vi "lookup_node_predecessors.vi"(10 "node":refnum<class "Node.lvclass">, 11 "digraph":refnum<class "DiGraph.lvclass">) -> (1 "predecessors":refnum<class "Node.lvclass">[](array[class]), 2 "node not found?":bool)   [LabVIEW 2020, in "graph.lvlib" / "DiGraph.lvclass"]
uses:
  DiGraph.lvclass
  C:/Projects/labview-project-load-tools/source/submodules/graph-api-labview/source/api/Graph/Graph.lvclass
  Node/Node.lvclass
  Node/Node.lvclass/Node.ctl
  DiGraph.lvclass/DiGraph.ctl
  Graph/Graph.lvclass/Graph.ctl
  Graph/Graph.lvclass
  0d9acaa0-7633-4a41-a63c-eb8e9d282815.vi
  C:/Projects/labview-project-load-tools/source/submodules/graph-api-labview/source/api/DiGraph/DiGraph.lvclass
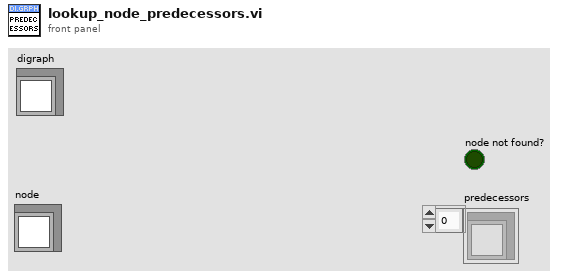
[diagram p1: front panel]
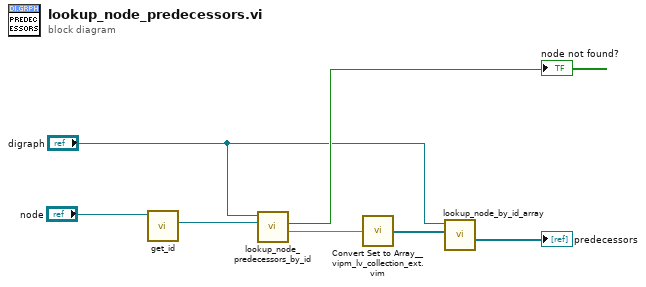
[diagram p0: block diagram]
diagram:
  n1 = call "get_id.vi"("node"="node") -> ("node-id"=w5:refnum<class "ID.lvclass">)  [unwired: 10 in]
  n2 = call "lookup_node_predecessors_by_id.vi"("node-id"=w5, "Graph in"="digraph") -> ("predecessors"=w3:set{refnum<class "ID.lvclass">}, "node not found?"=→"node not found?":bool)  [unwired: 8 in]
  n3 = call "Convert Set to Array__vipm_lv_collection_ext.vim"("set"=w3) -> ("array"=w4:refnum<class "ID.lvclass">[])  [unwired: 8 in]
  n4 = call "lookup_node_by_id_array.vi"("node_ids"=w4, "graph"="digraph") -> ("nodes"=→"predecessors":refnum<class "Node.lvclass">[])  [unwired: 8 in, 1 out]
